vi "get_settings_cluster.vi"(8 "error in (no error)":errorcluster, 11 "StimulatorDL090727DAQmx in":refnum<class "StimulatorDL090727Writer.lvclass">) -> (0 "error out":errorcluster, 2 "settings cluster":variant, 3 "StimulatorDL090727DAQmx out":refnum<class "StimulatorDL090727Writer.lvclass">)   [LabVIEW 2010, in "StimulatorDL090727Writer.lvclass"]
uses:
  StimulatorDL090727Writer.lvclass
  StimulatorDL090727Writer.lvclass/StimulatorDL090727Writer.ctl
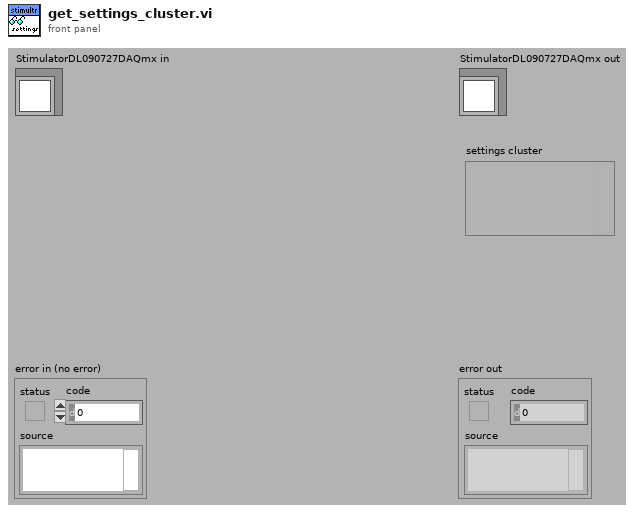
[diagram p1: front panel]
types:
  T1 = typedef "StimulatorDL090727Writer.lvclass/settings_cluster.ctl" = cluster{"Duration":dbl[unit], "Offset":dbl[unit], "DutyCycle":dbl[unit], "Type":T2, "Repetitions":i32, "Frequency":dbl[unit], "Amplitude":dbl}
  T2 = typedef "StimulatorDL090727Writer.lvclass/pattern_enum.ctl" = enum16{"sine wave", "square"}
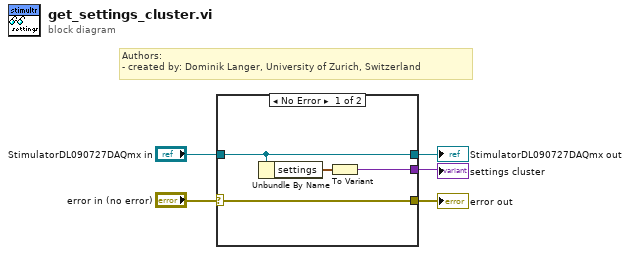
[diagram p0: block diagram]
diagram:
  # "Authors: \n- created by: Dominik Langer, University of Zurich, Switzerland"
  n1 = case shown="No Error" "error in (no error)" {
    selector: "error in (no error)" -> [w7 w11]
    tunnel: "StimulatorDL090727DAQmx in" -> [w6 w10]
    tunnel: [w8 _] -> w3
    tunnel: [w7 w11] -> w2
    tunnel: [w6 w10] -> w1
    frame No Error {
      n2 = Unbundle By Name(w6) -> ("settings"=w9:T1)
      n3 = To Variant(anything=w9) -> (Variant=w8:variant)
    }
    frame Error {
    }
  }
  "error out" <- w2
  "StimulatorDL090727DAQmx out" <- w1
  "settings cluster" <- w3
